vi "transform.vi"(8 "error in (no error)":errorcluster, 11 "Interface_transform in":refnum<class "Interface_transform.lvclass">) -> (0 "error out":errorcluster, 2 "X_new":dbl[][](array[numeric]), 3 "Interface_transform out":refnum<class "Interface_transform.lvclass">)   [LabVIEW 2020, in "Interface_transform.lvclass"]
doc: "Transform X."
uses:
  Interface_transform.lvclass
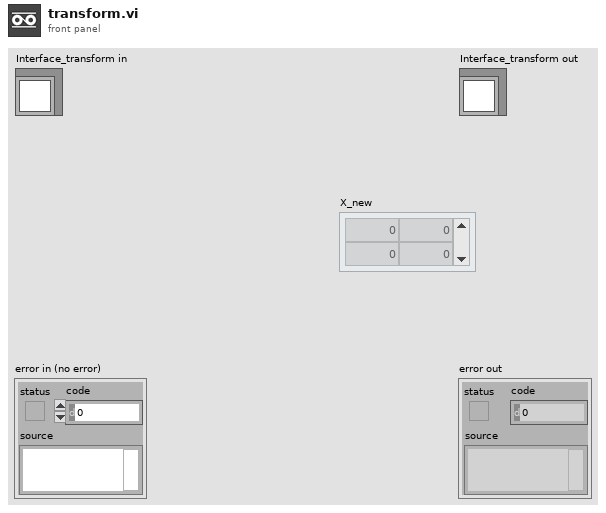
[diagram p1: front panel]
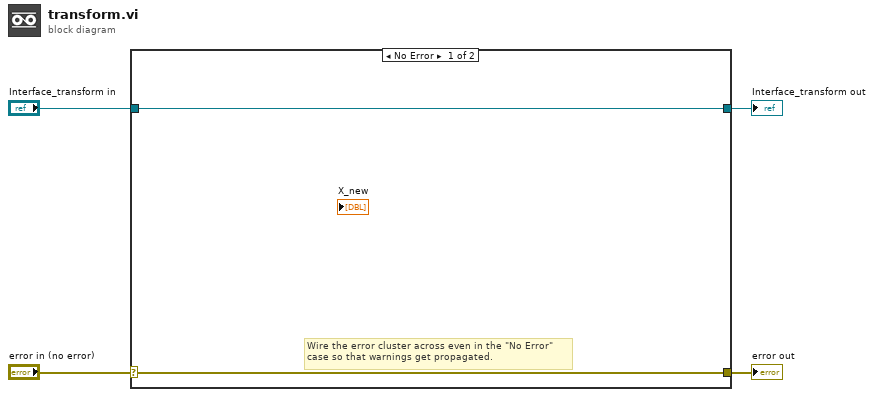
[diagram p0: block diagram]
diagram:
  n1 = case shown="No Error" "error in (no error)" {
    selector: "error in (no error)" -> [w5 w8]
    tunnel: [w5 w8] -> w3
    tunnel: [w6 w7] -> w1
    tunnel: "Interface_transform in" -> [w6 w7]
    frame No Error {
      # "Wire the error cluster across even in the \"No Error\"\ncase so that warnings get propagated."
    }
    frame Error {
    }
  }
  "error out" <- w3
  "Interface_transform out" <- w1
